vi "Create Enum Tables_Beltwatch.vi"() -> ()   [LabVIEW 2017, in "Copy of Beltwatch SQLite.lvlib"]
uses:
  Copy of Beltwatch SQLite.lvlib
  Common64/Database/SQ Lite/SQ Lite Cluster Action.ctl
  Beltwatch/SourceCode/BeltWatch Event type.ctl
  Beltwatch/SourceCode/BeltWatch Alarm Priority.ctl
  Beltwatch/SourceCode/Events class.ctl
panel:
  in  "Events Class":T1
  in  "Alarm priority":T2
  in  "Type":T3
  in  "Pre String":string="DROP TABLE IF EXISTS events;\n\n\nCREATE TABLE events (\n  db_id INTEGER PRIMARY KEY\n\n"
  in  "Readingse":T4[](array[typedef])=[{"Include"=TRUE, "Name"="Reading #", "SQLite3 type"=enum."SQLITE_INTEGER"}, {"Include"=TRUE, "Name"="Readings", "SQLite3 type"=enum."SQLITE3_TEXT"}, {"Include"=TRUE, "Name"="Reading Name", "SQLite3 type"=enum."SQLITE3_TEXT"}, {"Include"=TRUE, "Name"="TypeVal", "SQLite3 type"=enum."SQLITE_INTEGER"}, {"Include"=TRUE, "Name"="Alarm priority", "SQLite3 type"=enum."SQLITE_INTEGER"}, {"Include"=FALSE, "Name"="Display precision", "SQLite3 type"=enum."undefined type (0)"}, {"Include"=TRUE, "Name"="TypeStr", "SQLite3 type"=enum."SQLITE3_TEXT"}, {"Include"=TRUE, "Name"="AlarmPriorityStr", "SQLite3 type"=enum."SQLITE3_TEXT"}]
  out "?":errorcluster
  out "String":string
  out "SQLite3 type":T5(ring)
  in  "Events":T4[](array[typedef])=[{"Include"=TRUE, "Name"="Position", "SQLite3 type"=enum."SQLITE_INTEGER"}, {"Include"=TRUE, "Name"="Event Type", "SQLite3 type"=enum."SQLITE_INTEGER"}, {"Include"=TRUE, "Name"="Area", "SQLite3 type"=enum."SQLITE_INTEGER"}, {"Include"=TRUE, "Name"="Channels", "SQLite3 type"=enum."SQLITE_INTEGER"}, {"Include"=TRUE, "Name"="Start position", "SQLite3 type"=enum."SQLITE_INTEGER"}, {"Include"=TRUE, "Name"="End  position", "SQLite3 type"=enum."SQLITE_INTEGER"}, {"Include"=TRUE, "Name"="Name", "SQLite3 type"=enum."SQLITE3_TEXT"}, {"Include"=TRUE, "Name"="Offset", "SQLite3 type"=enum."SQLITE_INTEGER"}, {"Include"=TRUE, "Name"="Length", "SQLite3 type"=enum."SQLITE_INTEGER"}, {"Include"=FALSE, "Name"="Action marker", "SQLite3 type"=enum."undefined type (0)"}, {"Include"=TRUE, "Name"="Event", "SQLite3 type"=enum."SQLITE_INTEGER"}, {"Include"=TRUE, "Name"="# Defects", "SQLite3 type"=enum."SQLITE_INTEGER"}, {"Include"=TRUE, "Name"="jpg Image", "SQLite3 type"=enum."SQLITE_BLOB"}, {"Include"=FALSE, "Name"="chan maxs", "SQLite3 type"=enum."undefined type (0)"}, {"Include"=FALSE, "Name"="chan mins", "SQLite3 type"=enum."undefined type (0)"}, {"Include"=TRUE, "Name"="TimeStamp", "SQLite3 type"=enum."SQLITE_INTEGER"}, {"Include"=TRUE, "Name"="Readings", "SQLite3 type"=enum."SQLITE_INTEGER"}, {"Include"=TRUE, "Name"="ID", "SQLite3 type"=enum."SQLITE_INTEGER"}, {"Include"=TRUE, "Name"="New", "SQLite3 type"=enum."SQLITE_INTEGER"}, {"Include"=FALSE, "Name"="Hires Track", "SQLite3 type"=enum."undefined type (0)"}, {"Include"=FALSE, "Name"="2D overlay", "SQLite3 type"=enum."undefined type (0)"}, {"Include"=FALSE, "Name"="update", "SQLite3 type"=enum."undefined type (0)"}, {"Include"=TRUE, "Name"="Field #", "SQLite3 type"=enum."SQLITE_INTEGER"}, {"Include"=TRUE, "Name"="Events Class", "SQLite3 type"=enum."SQLITE_INTEGER"}, {"Include"=FALSE, "Name"="Sync", "SQLite3 type"=enum."undefined type (0)"}, {"Include"=TRUE, "Name"="Insert Offset", "SQLite3 type"=enum."SQLITE_INTEGER"}, {"Include"=TRUE, "Name"="Next trend", "SQLite3 type"=enum."SQLITE_INTEGER"}, {"Include"=TRUE, "Name"="Speed", "SQLite3 type"=enum."SQLITE_INTEGER"}]
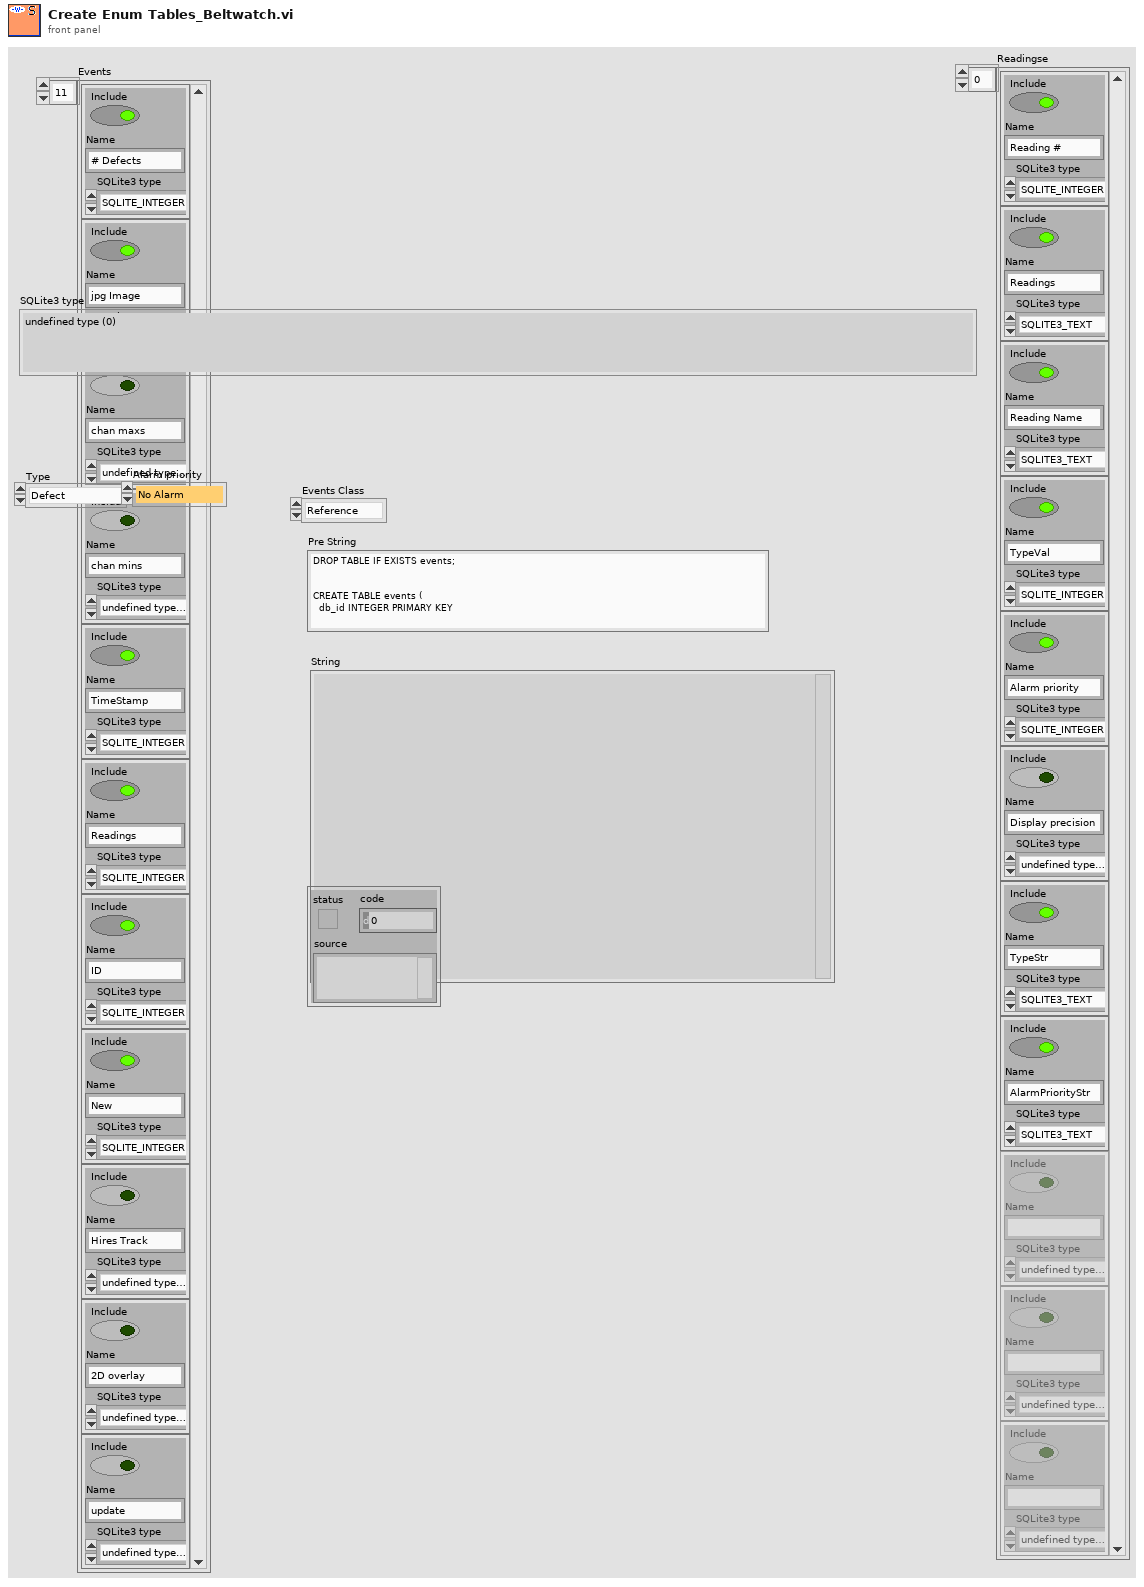
[diagram p1: front panel]
types:
  T1 = typedef "Events class.ctl" = enum16{"Reference", "Inspection", "New", "Tramp", "Align", "Ready"}
  T2 = typedef "BeltWatch Alarm Priority.ctl" = enum16{"No Alarm", "High", "Medium", "Low"}
  T3 = typedef "BeltWatch Event type.ctl" = enum16{"Defect", "Splice", "Break", "Rip", "Track", "Segment", "Belt", "New Splice", "Missing Splice", "None", "Free"}
  T4 = typedef "Copy of Beltwatch SQLite.lvlib/SQ Lite Cluster Action.ctl" = cluster{"Include":bool, "Name":string, "SQLite3 type":enum32{"undefined type (0)", "SQLITE_INTEGER", "SQLITE_FLOAT", "SQLITE3_TEXT", "SQLITE_BLOB", "SQLITE_NULL", "undefined type", "FloatArray"}}
  T5 = enum32{"undefined type (0)", "SQLITE_INTEGER", "SQLITE_FLOAT", "SQLITE3_TEXT", "SQLITE_BLOB", "SQLITE_NULL", "undefined type"}
  T6 = enum32{"undefined type (0)", "SQLITE_INTEGER", "SQLITE_FLOAT", "SQLITE3_TEXT", "SQLITE_BLOB", "SQLITE_NULL", "undefined type", "FloatArray"}
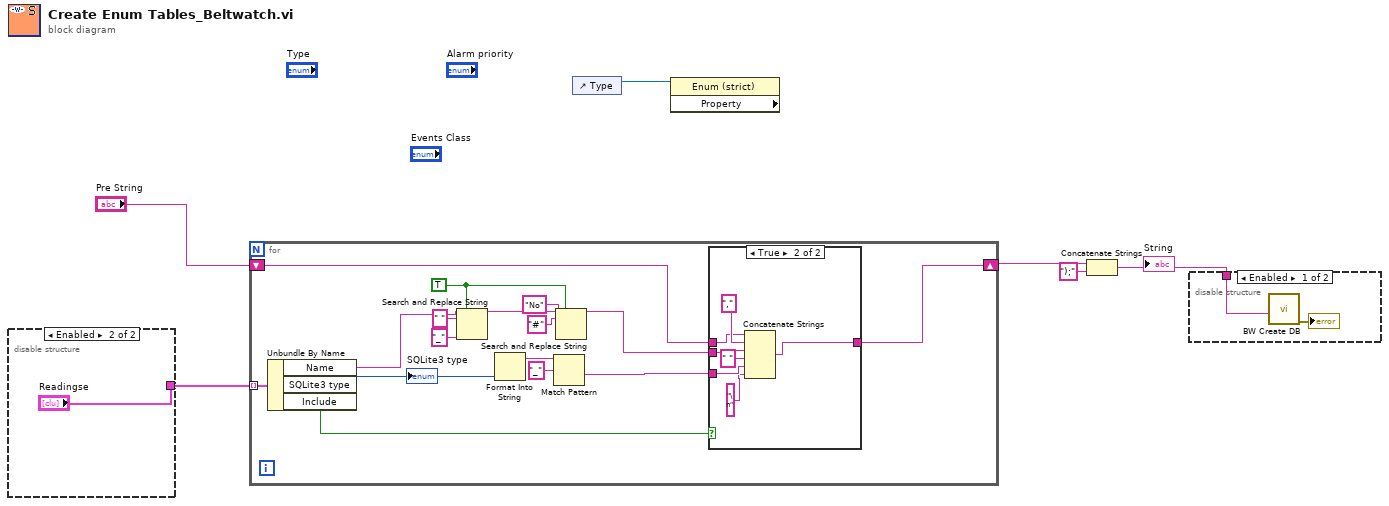
[diagram p0: block diagram]
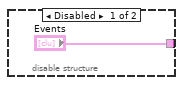
[diagram p2: hidden frame]
diagram:
  n1 = disable-structure shown="Enabled" {
    disable-tunnel: ["Events" "Readingse"] -> w5
    frame Disabled {
    }
    frame Enabled {
    }
  }
  n2 = for {
    shift-right: [w17] -> w4
    shift-left: "Pre String" -> [w24]
    tunnel: w5 -> [w23] mode=indexing
    w13 = TRUE ("replace all? (F)")
    n3 = Unbundle By Name(w23) -> ("Name"=w16:string, "SQLite3 type"=w21:T6, "Include"=w22:bool)
    "SQLite3 type" <- w21
    n4 = Search and Replace String(replace all?=w13, input string=w16, search string=" ", replace string="_" ("replace string (\"\")")) -> (result string=w12:string)  [unwired: 4 in, 3 out]
    n5 = Format Into String(w21) -> (resulting string=w20:string)  [unwired: 3 in, 1 out]
    n6 = Match Pattern(string=w20, regular expression="_") -> (after substring=w18:string)  [unwired: 1 in, 3 out]
    n7 = Search and Replace String(replace all?=w13, input string=w12, search string="#" ("replace string (\"\")"), replace string="No" ("replace string (\"\")")) -> (result string=w9:string)  [unwired: 4 in, 3 out]
    n8 = case shown="True" w22 {
      tunnel: w24 -> [w25 w27]
      tunnel: w9 -> [_ w32]
      tunnel: w18 -> [_ w30]
      tunnel: [w25 w29] -> w17
      frame False {
      }
      frame True {
        n9 = Concatenate Strings(w27, "," ("string"), w32, " " ("string"), w30, "\n" ("string")) -> (w29:string)
      }
    }
  }
  n10 = control-ref of="Type"() -> (w1:refnum<vi>)
  n11 = property class="Enum (strict)" props=[](reference=w1) -> ()  [unwired: 1 in, 3 out]
  n12 = Concatenate Strings(w4, ");" ("string")) -> (w2:string)
  "String" <- w2
  n13 = disable-structure shown="Enabled" {
    disable-tunnel: w2 -> [w34 _]
    frame Enabled {
      n14 = call "BW Create DB.vi"("String"=w34) -> ("error out"=→"?":errorcluster)  [unwired: 10 in]
    }
    frame Disabled {
    }
  }
